vi "LinkNodes.vi"(6 "index":i32, 8 "error in":errorcluster, 10 "child in":T1, 11 "parent in":T1) -> (0 "error out":errorcluster, 2 "child out":T1, 3 "parent out":T1)   [LabVIEW 2013, in "NISE_CEF_Node.lvclass"]
doc: "Links 2 nodes together one as a parent and one as a child."
uses:
  NISE_CEF_Node.lvclass
  NodeRef.ctl
  NISE_CEF_Node.lvclass/NISE_CEF_Node.ctl
  ReadChildren.vi
  WriteChildren.vi
  WriteParent.vi
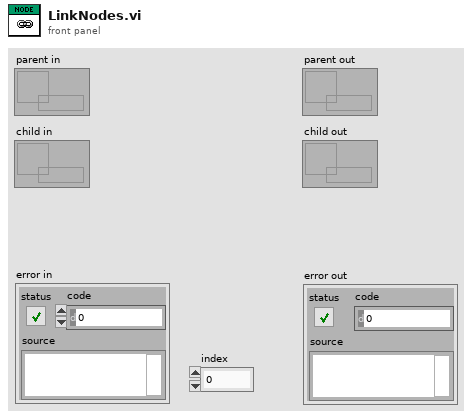
[diagram p1: front panel]
types:
  T1 = typedef "NISE_CEF_Node.lvclass/NodeRef.ctl" = refnum<data-value>
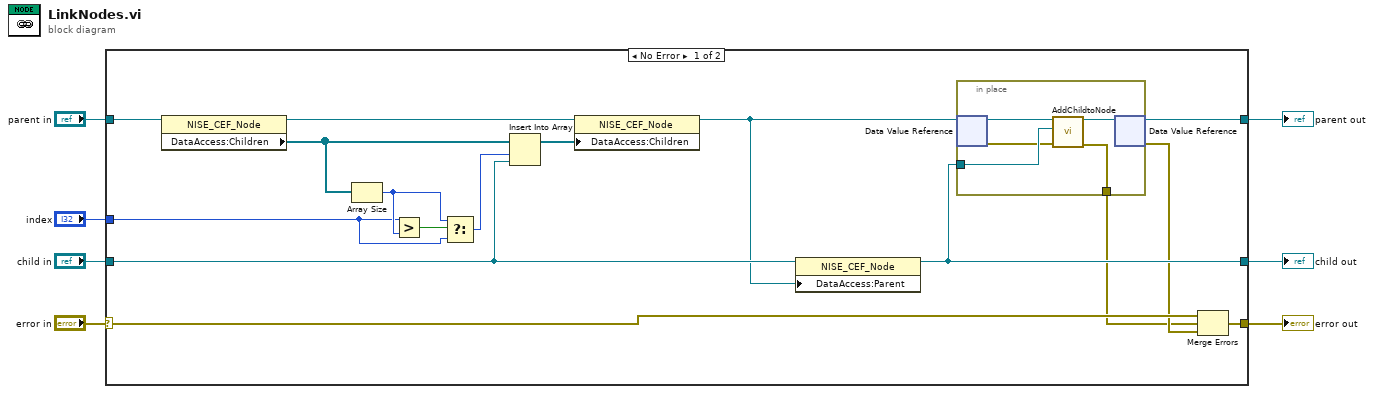
[diagram p0: block diagram]
diagram:
  n1 = case shown="No Error" "error in" {
    selector: "error in" -> [w23 w31]
    tunnel: [w10 w31] -> w3
    tunnel: "parent in" -> [w17 w30]
    tunnel: "child in" -> [w14 w29]
    tunnel: [w12 w29] -> w2
    tunnel: [w11 w30] -> w1
    tunnel: "index" -> [w20 _]
    frame No Error {
      n2 = property class="NISE_CEF_Node"(reference=w17) -> (reference out=w15:T1, "DataAccess:Children"=w19:T1[])  [unwired: 1 in, 1 out]
      n3 = Array Size(array=w19) -> (size(s)=w21:i32)
      n4 = Greater?(x=w20, y=w21) -> (0:w22:bool)
      n5 = Select(t=w21, s=w22, f=w20) -> (s? t:f=w18:i32)
      n6 = Insert Into Array(array=w19, index=w18, new element=w14) -> (w16:T1[])
      n7 = property class="NISE_CEF_Node"(reference=w15, "DataAccess:Children"=w16) -> (reference out=w13:T1)  [unwired: 1 in, 1 out]
      n8 = property class="NISE_CEF_Node"(reference=w14, "DataAccess:Parent"=w13) -> (reference out=w12:T1)  [unwired: 1 in, 1 out]
      n9 = in-place {
        in-place-border: w12 -> [w26]
        in-place-border: [w24] -> w8
        n10 = in-place-dvr #1(w13) -> (w28:refnum<class "NISE_CEF_Node.lvclass">, w25:errorcluster)
        n11 = call-dynamic "AddChildtoNode.vi"("error in"=w25, "child in"=w26, "NISE_CEF_Node in"=w28) -> ("error out"=w24:errorcluster, "NISE_CEF_Node out"=w27:refnum<class "NISE_CEF_Node.lvclass">)  [unwired: 7 in]
        n12 = in-place-dvr #1(w27) -> (w11:T1, w9:errorcluster)
      }
      n13 = Merge Errors(w23, w8, w9) -> (w10:errorcluster)
    }
    frame Error {
    }
  }
  "error out" <- w3
  "child out" <- w2
  "parent out" <- w1
